vi "Actor Core.vi"(8 "error in":errorcluster, 11 "Nested in":refnum<class "CallActorCenter.lvclass">) -> (0 "error out":errorcluster, 3 "Actor out":refnum<class "Actor.lvclass">)   [LabVIEW 2021, in "CallActorCenter.lvclass"]
doc: "(<B>Filename</B>: Actor Framework.lvlib:Actor.lvclass:Actor Core.vi)\n\nReceives messages to the actor, reacts to them, and initiates any error handling that may shut the actor down.\n\nDescendant classes may override this VI to append parallel tasks for the actor to complete while it handles messages. Overrides use the Call Parent Method node."
uses:
  CallActorCenter.lvclass
  CallActorCenter.lvclass/CallActorCenter.ctl
  <userlib>/John_Lib/AbstractActorTemplate/AbstractActorTemplate/UIActorTop.lvclass
  C:/Program Files (x86)/National Instruments/LabVIEW 2021/user.lib/John_Lib/AbstractActorTemplate/AbstractActorTemplate/UIActorTop.lvclass
  C:/Program Files (x86)/National Instruments/LabVIEW 2021/vi.lib/ActorFramework/Actor/Actor.lvclass
  C:/Program Files (x86)/National Instruments/LabVIEW 2021/project/Create Actor from Template/_ActorCenter/CallActorCenter.lvclass
  C:/Program Files (x86)/National Instruments/LabVIEW 2021/user.lib/John_Lib/Interfaces/InsertLeftSubPanel/InsertLeftSubPanel.lvclass
  C:/Program Files (x86)/National Instruments/LabVIEW 2021/user.lib/John_Lib/Interfaces/InsertMainSubPanel/InsertMainSubPanel.lvclass
  C:/Program Files (x86)/National Instruments/LabVIEW 2021/user.lib/John_Lib/Interfaces/InsertRightSubPanel/InsertRightSubPanel.lvclass
  <vilib>/ActorFramework/Actor/Actor.lvclass
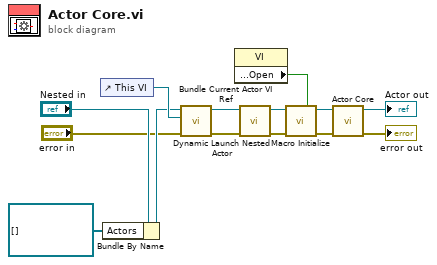
[diagram p0: block diagram]
diagram:
  n1 = control-ref of="This VI"() -> (w5:refnum<vi>)
  n2 = Bundle By Name(cluster="Nested in", "Actors"=refnum<class "UIActorTop.lvclass">[] []) -> (w4:refnum<class "CallActorCenter.lvclass">)
  n3 = call <userlib>:"Bundle Current Actor VI Ref.vi"("error in (no error)"="error in", "This VI"=w5, "UI ActorTop in"=w4) -> ("error out"=w6:errorcluster, "UI ActorTop in"=w7:refnum<class "CallActorCenter.lvclass">)  [unwired: 6 in, 1 out]
  n4 = property class="VI"() -> ("Front Panel.Open"=w11:bool)  [unwired: 2 in, 2 out]
  n5 = call-dynamic "Dynamic Launch Nested Actor.vi"("error in (no error)"=w6, "UI ActorTop in"=w7) -> ("error out"=w12:errorcluster, "UI ActorTop out"=w13:refnum<class "CallActorCenter.lvclass">)  [unwired: 8 in]
  n6 = call-dynamic "Macro Initialize.vi"("Front Panel Window:Open"=w11, "error in (no error)"=w12, "UI ActorTop in"=w13) -> ("error out"=w9:errorcluster, "UI ActorTop out"=w10:refnum<class "CallActorCenter.lvclass">)  [unwired: 7 in]
  n7 = call-parent "Actor Core.vi"("error in"=w9, "Actor in"=w10) -> ("error out"=→"error out":errorcluster, "Actor out"=→"Actor out":refnum<class "Actor.lvclass">)  [unwired: 8 in]
